vi "tcp_sweep_preset.vi"(10 "points_in":string, 11 "freq_range":cluster{"start_freq":string, "stop_freq":string}) -> (1 "points_out":i32, 2 "stop_freq":dbl, 3 "start_freq":dbl)   [LabVIEW 2025]
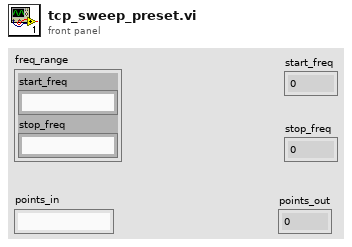
[diagram p1: front panel]
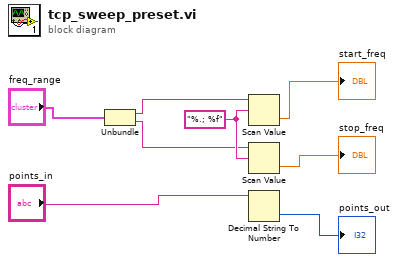
[diagram p0: block diagram]
diagram:
  w8 = "%.; %f" ("format string")
  n1 = Unbundle("freq_range") -> ("start_freq"=w4:string, "stop_freq"=w3:string)
  n2 = Scan Value(string=w4, format string=w8) -> (value=→"start_freq":dbl)  [unwired: 1 in, 1 out]
  n3 = Scan Value(string=w3, format string=w8) -> (value=→"stop_freq":dbl)  [unwired: 1 in, 1 out]
  n4 = Decimal String To Number(string="points_in") -> (number=→"points_out":i32)  [unwired: 2 in, 1 out]
